vi "FailureDescription.vi"(8 "error in (no error)":errorcluster, 10 "Actual":variant, 11 "Is Same Type in":refnum<class "Is Same Type.lvclass">) -> (0 "error out":errorcluster, 2 "Failure Description":string, 3 "Is Same Type out":refnum<class "Is Same Type.lvclass">)   [LabVIEW 2017, in "Transparent Assertions.lvlib" / "Constraints.lvlib" / "Is Same Type.lvclass"]
doc: "Return the second part of the scentence \"Failed asserting that ...\""
uses:
  Is Same Type.lvclass
  <vilib>/Utility/Data Type/NI_Data Type.lvlib
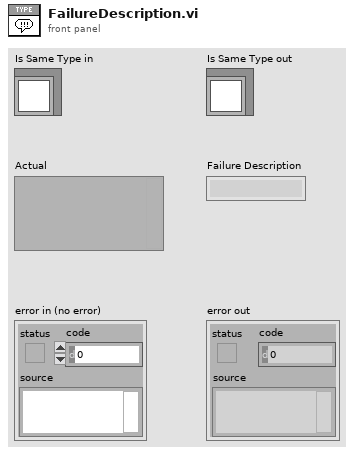
[diagram p1: front panel]
types:
  T1 = typedef "NI_Data Type.lvlib/Data Type.ctl" = enum8{"Invalid Type", "Void", "I8", "I16", "I32", "I64", "U8", "U16", "U32", "U64", "Single Float", "Double Float", "Extended Float", "Single Complex", "Double Complex", "Extended Complex", "Enum U8", "Enum U16", "Enum U32", "Enum U64", "Single Float With Unit", "Double Float With Unit", "Extended Float With Unit", "Single Complex with Unit", "Double Complex with Unit", "Extended Complex with Unit", "Boolean", "String", "Path", "Picture", "Tag", "Array", "Cluster", "Variant", "LV Variant", "Waveform", "Timestamp", "Digital Waveform", "Digital Data", "ExpressData", "Refnum", "External Data", "VI", "Poly VI", "LabVIEW Class Instance", "Fixed Point"}
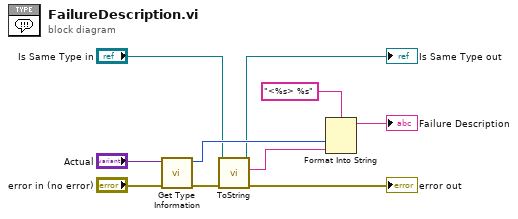
[diagram p0: block diagram]
diagram:
  n1 = call <vilib>:"Get Type Information.vi"("error in (no error)"="error in (no error)", "Variant"="Actual") -> ("error out"=w9:errorcluster, "Type"=w6:T1)  [unwired: 5 in, 3 out]
  n2 = call-dynamic "ToString.vi"("error in (no error)"=w9, "Is Same Type in"="Is Same Type in") -> ("error out"=→"error out":errorcluster, "String"=w3:string, "Is Same Type out"=→"Is Same Type out":refnum<class "Is Same Type.lvclass">)  [unwired: 7 in]
  n3 = Format Into String(format string="<%s> %s", w6, w3) -> (resulting string=→"Failure Description":string)  [unwired: 2 in, 1 out]
